vi "TestCloneAPI.vi"() -> ()   [LabVIEW 2018, in "AcPwrModule.lvlib"]
uses:
  AcPwrModule.lvlib
  AcPwrPlugins/ChromaAcLoad/TypeDefs/DeviceProperties.ctl
  TestInfo.ctl
  <userlib>/NIST/ModuleAdminLib/CloneRegistration/CloneRegistration.lvclass
  <userlib>/NIST/ModuleAdminLib/ModuleAdmin/ModuleAdmin.lvclass/ModuleAdmin.ctl
  <userlib>/NIST/ModuleAdminLib/ModuleAdmin/ModuleAdmin.lvclass
  PublicAPI/Arguments/Broadcasts/clDidInit.ctl
  PublicAPI/Arguments/Requests/clStopArgument.ctl
  <userlib>/NIST/ModuleAdminLib/ModuleAdmin/Accessors/Read CloneRegRef.vi
  <userlib>/NIST/ModuleAdminLib/ModuleAdmin/Accessors/Write CloneRegRef.vi
  AcPwrPlugins/AcPwrBaseClass/AcPwrBase.lvclass
  Visualization/Visualization.lvlib
  AcPwrPlugins/ChromaAcLoad/ChromaAcLoad.lvclass
panel:
  in  "Cluster":T1 {"Phases"."Phase Select" items=["Phase ALL", "Phase A", "Phase B", "Phase C"]}
  in  "btnSet":bool
  in  "btnGet":bool
  in  "btnVisualize":bool
  in  "Tab Control":enum32{"AC", "DC"}(tab)
  out "PacificPower":waveform(dbl)[](graph) caption="4140002"
  out "PP Incorrect Data Type?":bool
  out "Chroma AC":waveform(dbl)[](graph) caption="4140002"
  out "Chroma AC Incorrect Data Type?":bool
  out "NHRDC":waveform(sgl)[](graph) caption="4140002"
  out "NHRDC Incorrect Data Type?":bool
  out "Chroma DC":waveform(dbl)[](graph) caption="4140002"
  out "Chroma DC Incorrect Data Type?":bool
  in  "PP Program Number":i32=1 min=1 max=99
  in  "btnInitialize":bool
  in  "btnClearStatusLog":bool
  in  "btnDeviceOff":bool
  in  "btnDeviceOn":bool
  in  "btnConfigDevice":bool caption="btnConfigDevices"
  in  "btnStartMeas":bool
  in  "btnStopMeas":bool
  in  "btnClose":bool
  in  "btnReset":bool
  in  "btnPref":bool
  in  "Show Panel":bool
  in  "Plugin Type":u16(ring) items=["AcPwrBase", "ChromaDCLoad", "ChromaACLoad", "NHRDCPower", "PPS360AMXT"]
  in  "btnLoadPlugin":bool
  out "Path":path
  in  "btnRequestINIPath":bool
  in  "btnRemove":bool
  out "Status Log":string
  out "Active Modules (Array)":string[](array[string])
  in  "btnAdd":bool
  in  "btnStop":bool
  in  "Select Module":i32(ring)=-1 caption="Select Module to send Request" items=["All"=-1]
  # "Measurements"
  # "Hidden"
  # "Visible"
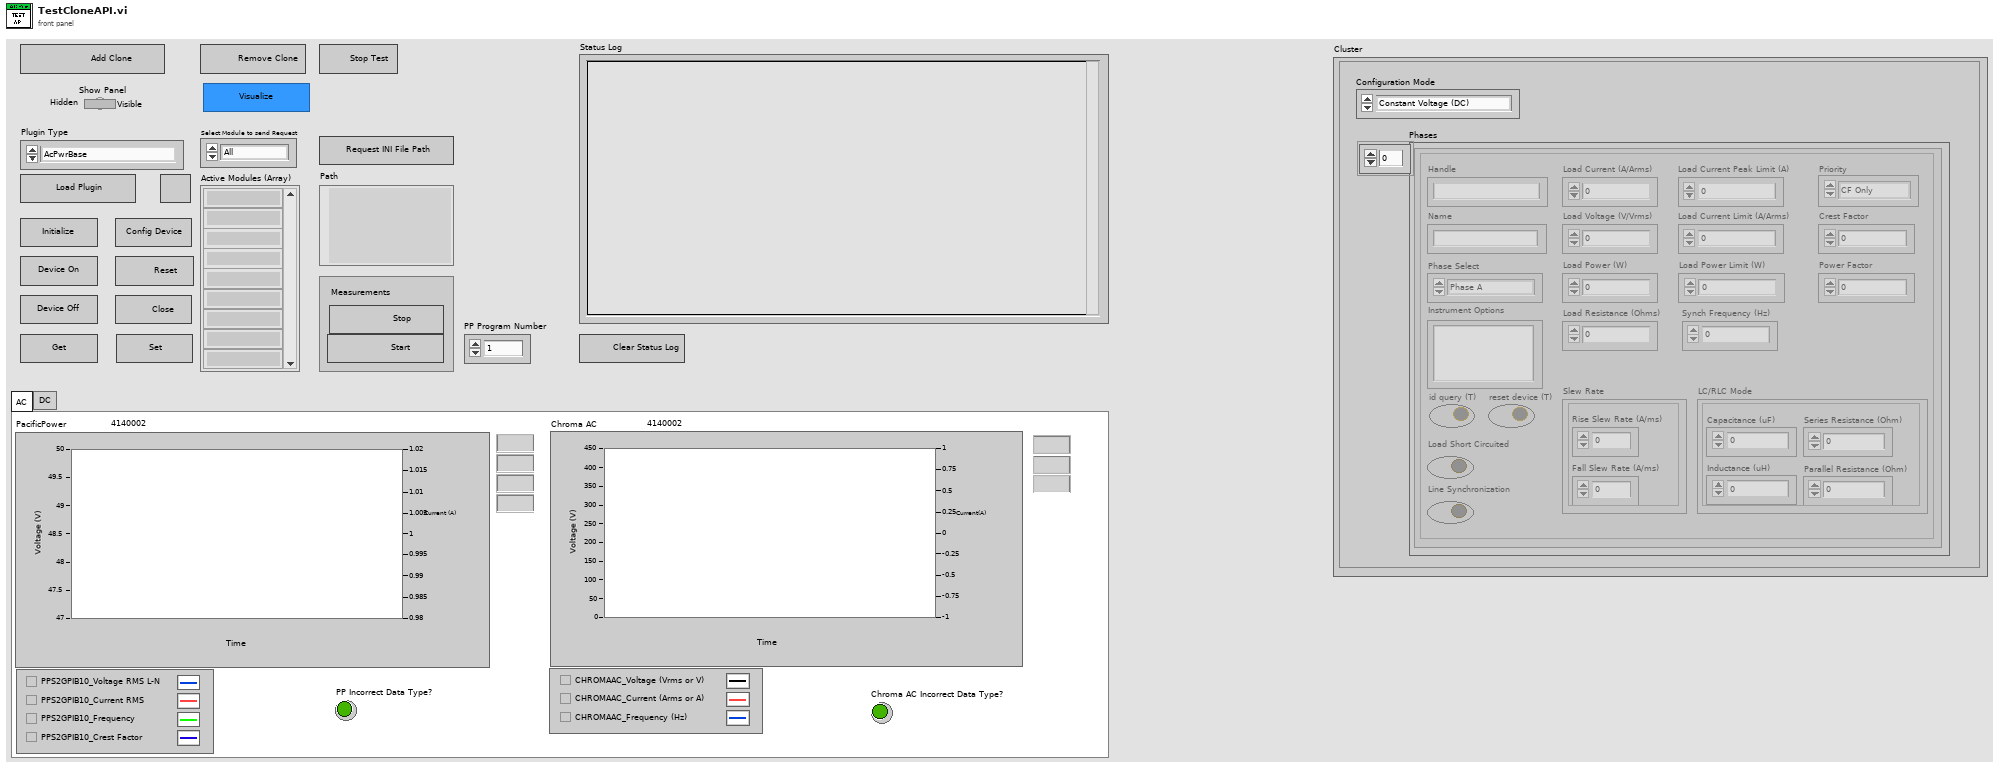
[diagram p1: front panel]
types:
  T1 = typedef "AcPwrPlugins.lvlib/ChromaAcLoad.lvclass/DeviceProperties.ctl" = cluster{"Configuration Mode":enum16{"Constant Voltage (DC)", "Constant Power (DC)", "Constant Power (AC)", "Constant Current (DC)", "Constant Current (AC)", "Constant Resistance (DC)", "Constant Resistance (AC)", "Rectified Mode (DC)", "Inrush (AC)", "RLC CP (AC)", "RLC (AC)"}, "Phases":cluster{"Handle":string, "Name":string, "Phase Select":i32, "Instrument Options":string, "id query (T)":bool, "reset device (T)":bool, "Load Short Circuited":bool, "Line Synchronization":bool, "Load Current (A/Arms)":dbl, "Load Voltage (V/Vrms)":dbl, "Load Power (W)":dbl, "Load Resistance (Ohms)":dbl, "Load Current Peak Limit (A)":dbl, "Load Current Limit (A/Arms)":dbl, "Load Power Limit (W)":dbl, "Synch Frequency (Hz)":dbl, "Priority":enum16{"CF Only", "PF Only", "Both (CF)", "Both (PF)"}, "Crest Factor":dbl, "Power Factor":dbl, "Slew Rate":cluster{"Rise Slew Rate (A/ms)":i32, "Fall Slew Rate (A/ms)":i32}, "LC/RLC Mode":cluster{"Capacitance (uF)":i32, "Inductance (uH)":i32, "Series Resistance (Ohm)":dbl, "Parallel Resistance (Ohm)":dbl}, "Timing":cluster{"TimingOn":enum16{""}, "Hours":u32, "Minutes":u32, "Seconds":dbl, "CutoffVoltage":dbl}, "Connected":bool}[]}
  T2 = typedef "AcPwrModule.lvlib/TestInfo.ctl" = cluster{"PluginIniFilePaths":path[]}
  T3 = typedef "AcPwrModule.lvlib/clBroadcastEvents.ctl" = cluster{"DidInit":refnum<user-event>, "StatusUpdate":refnum<user-event>, "ErrorReport":refnum<user-event>, "DidStop":refnum<user-event>, "PathToINI":refnum<user-event>, "Measurements":refnum<user-event>, "LoadConfigFile":refnum<user-event>, "GetSettings":refnum<user-event>, "SetSettings":refnum<user-event>, "GetType&ID":refnum<user-event>}
  T4 = typedef "AcPwrModule.lvlib/clDidInit.ctl" = cluster{"Init?":bool, "ModuleAdmin":refnum<class "ModuleAdmin.lvclass">}
  T5 = typedef "AcPwrModule.lvlib/clStopArgument.ctl" = cluster{"Exit via Stop Module Req?":bool, "Wait for Module to stop?":bool, "ModuleAdmin":refnum<class "ModuleAdmin.lvclass">}
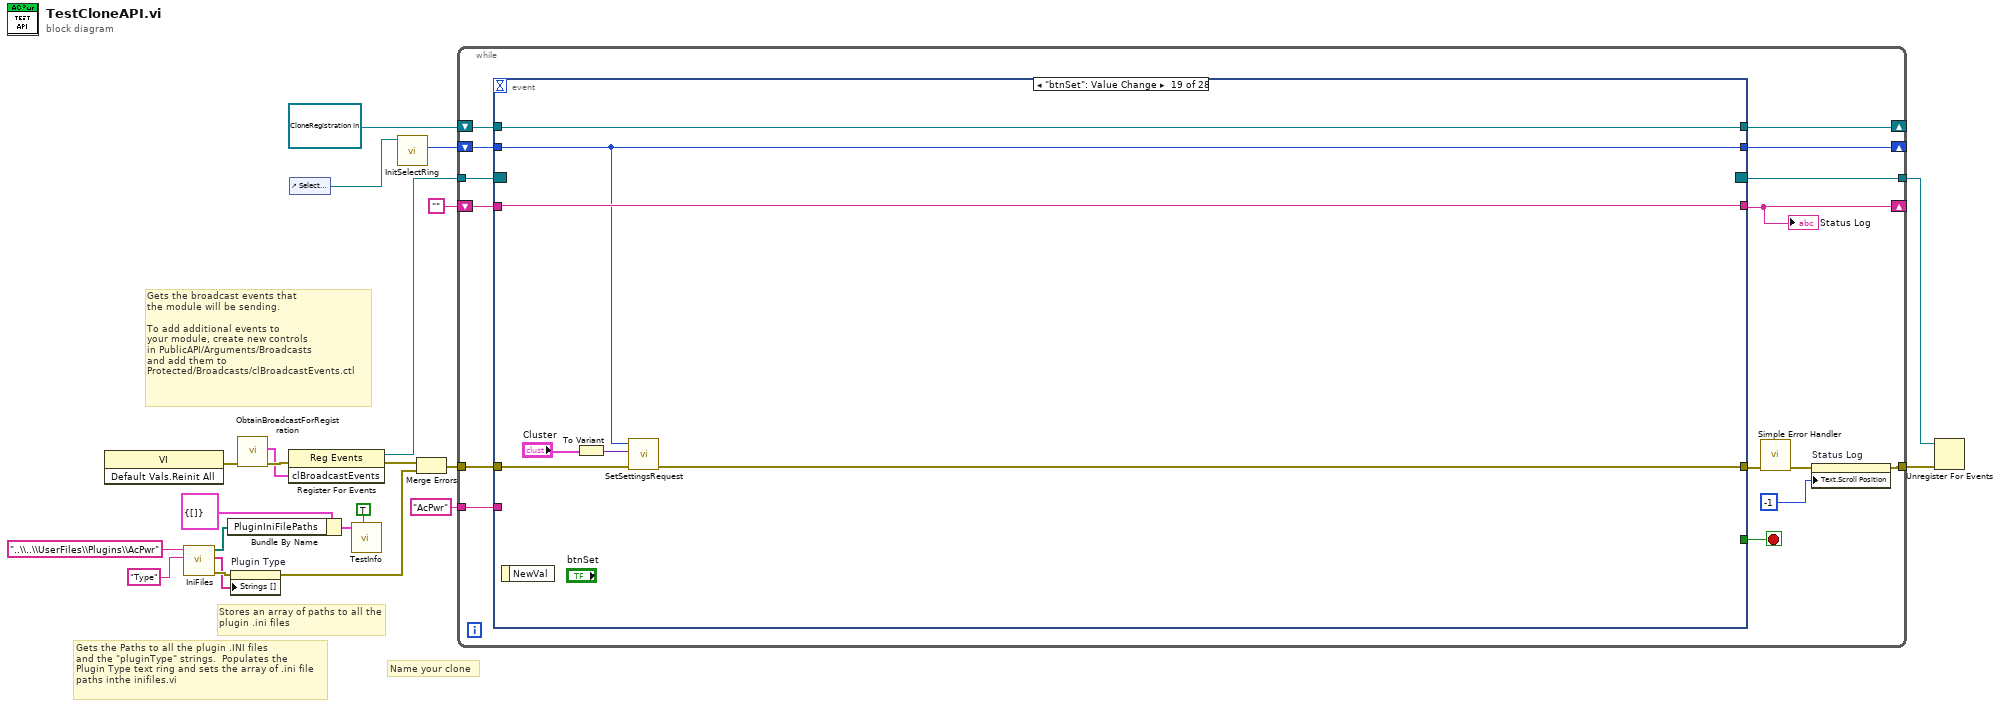
[diagram p0: block diagram]
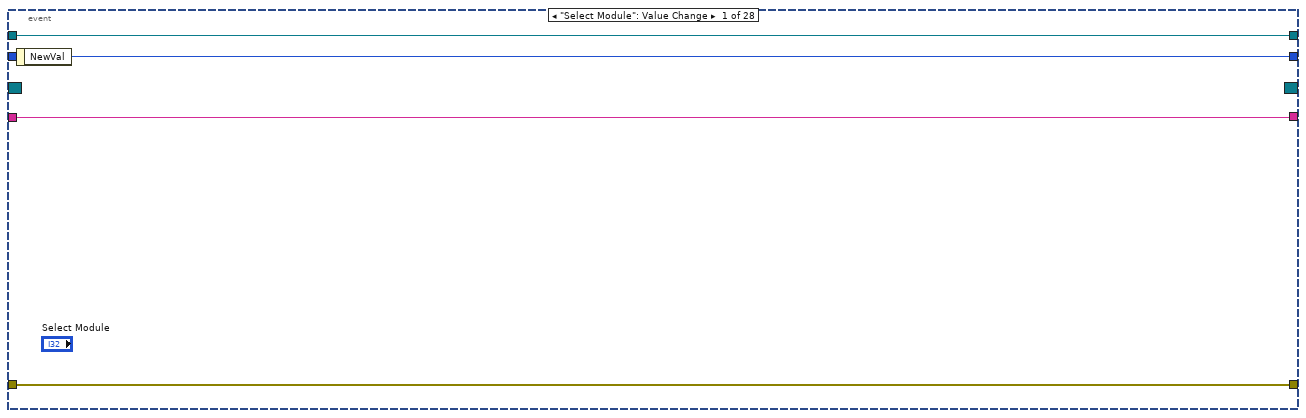
[diagram p2: hidden frame]
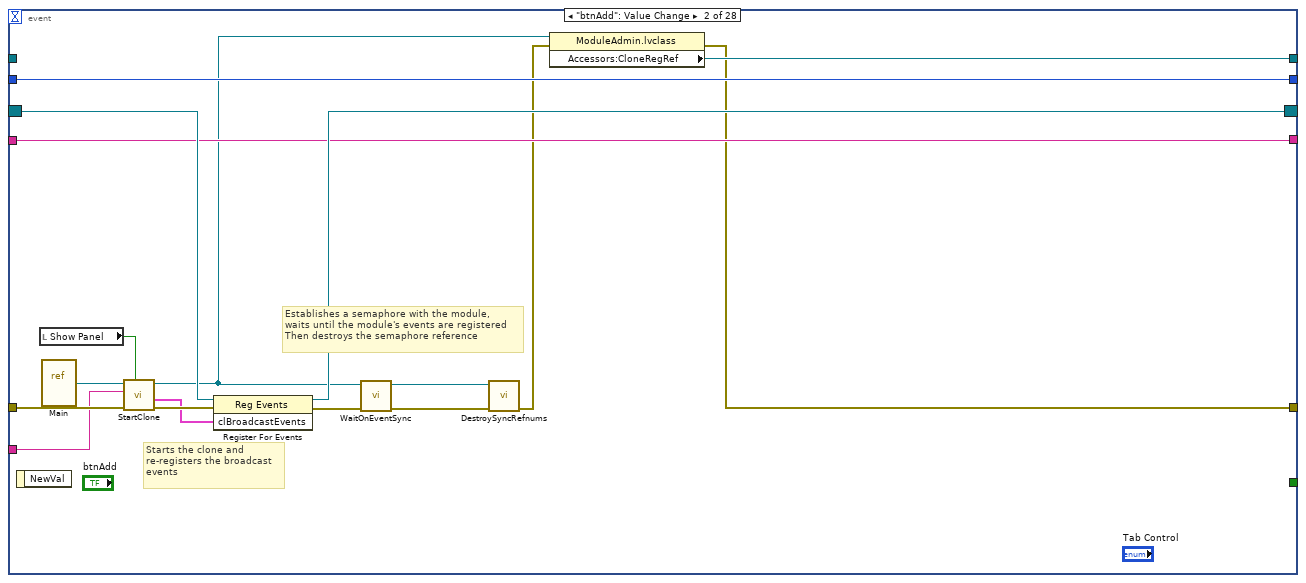
[diagram p3: hidden frame]
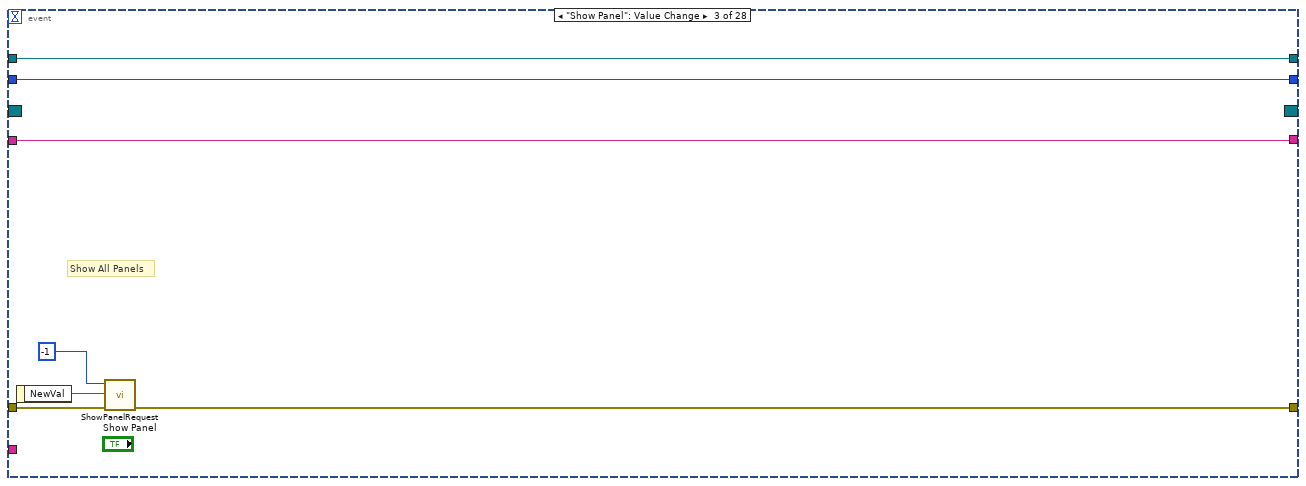
[diagram p4: hidden frame]
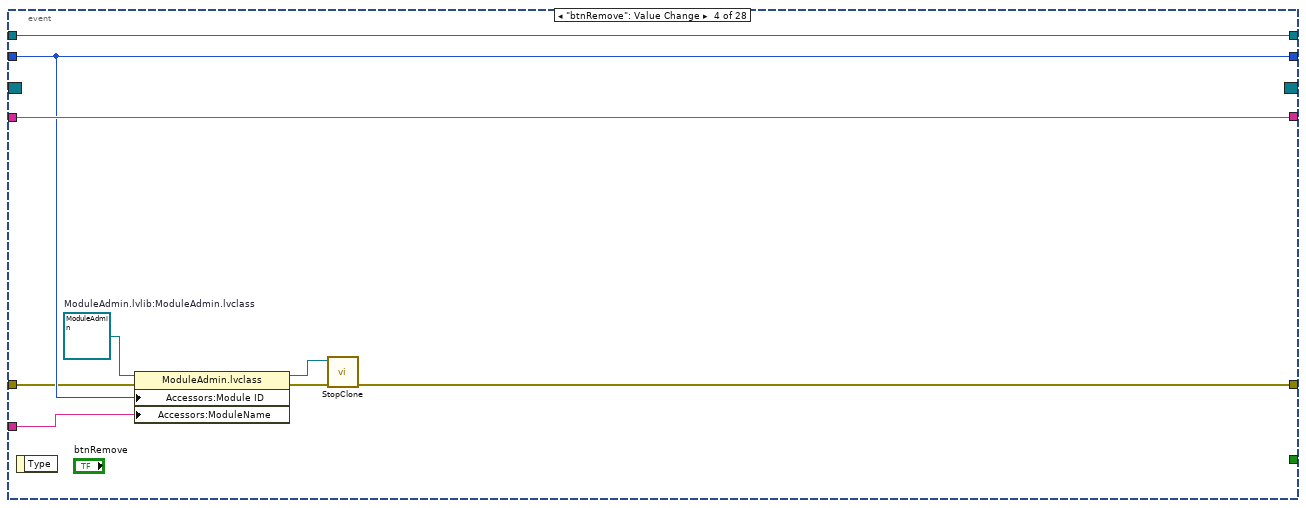
[diagram p5: hidden frame]
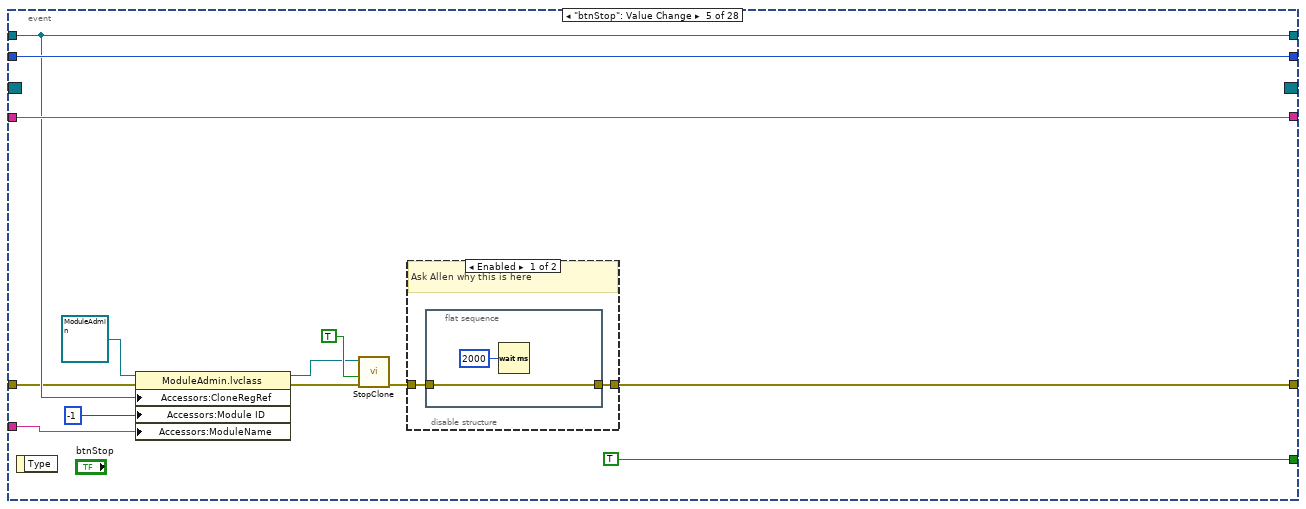
[diagram p6: hidden frame]
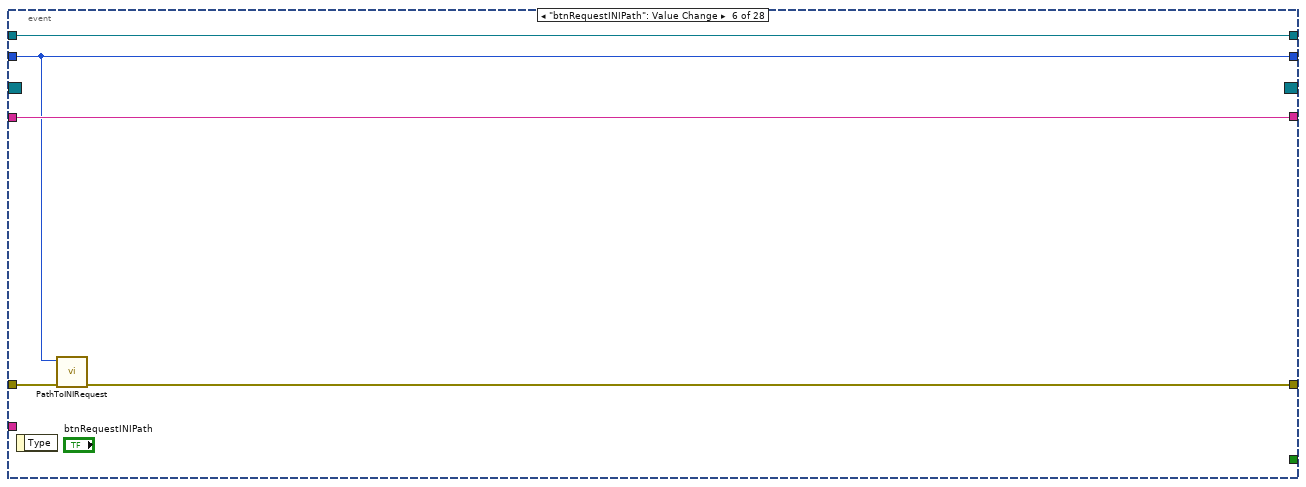
[diagram p8: hidden frame]
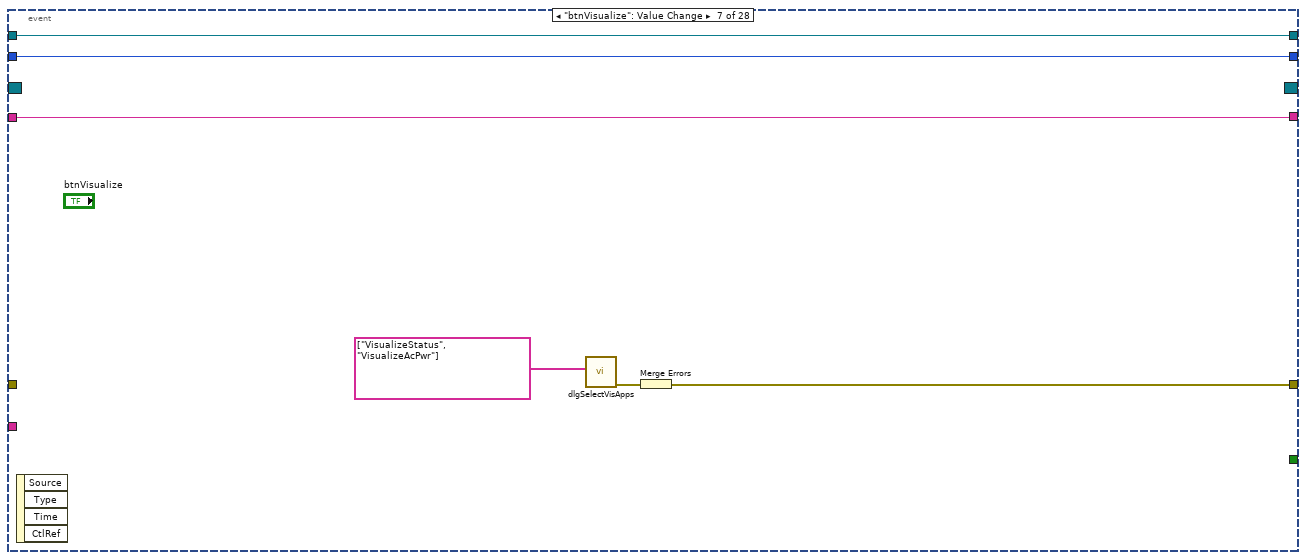
[diagram p9: hidden frame]
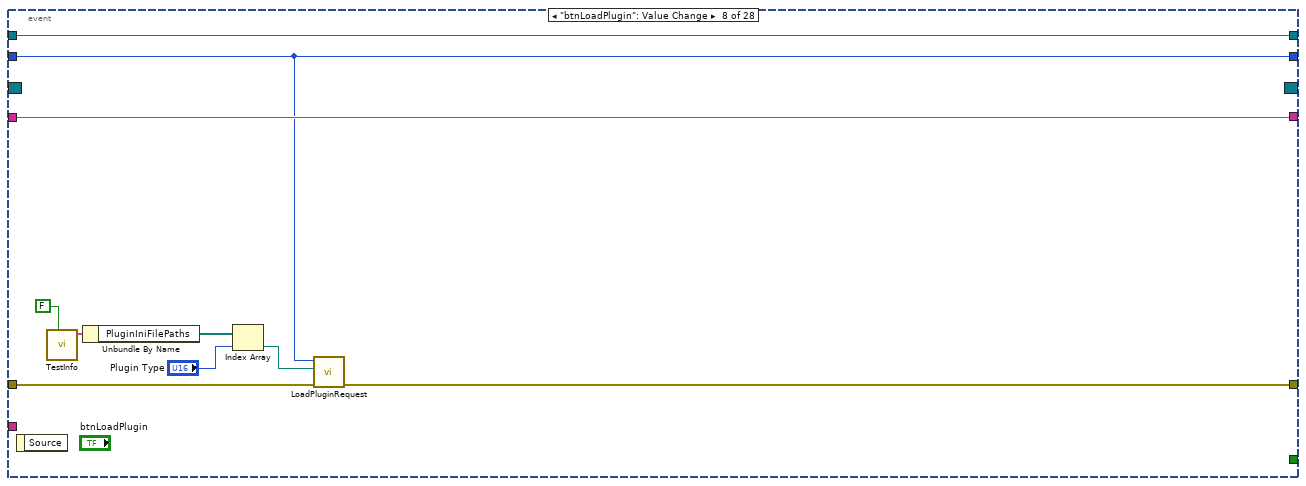
[diagram p10: hidden frame]
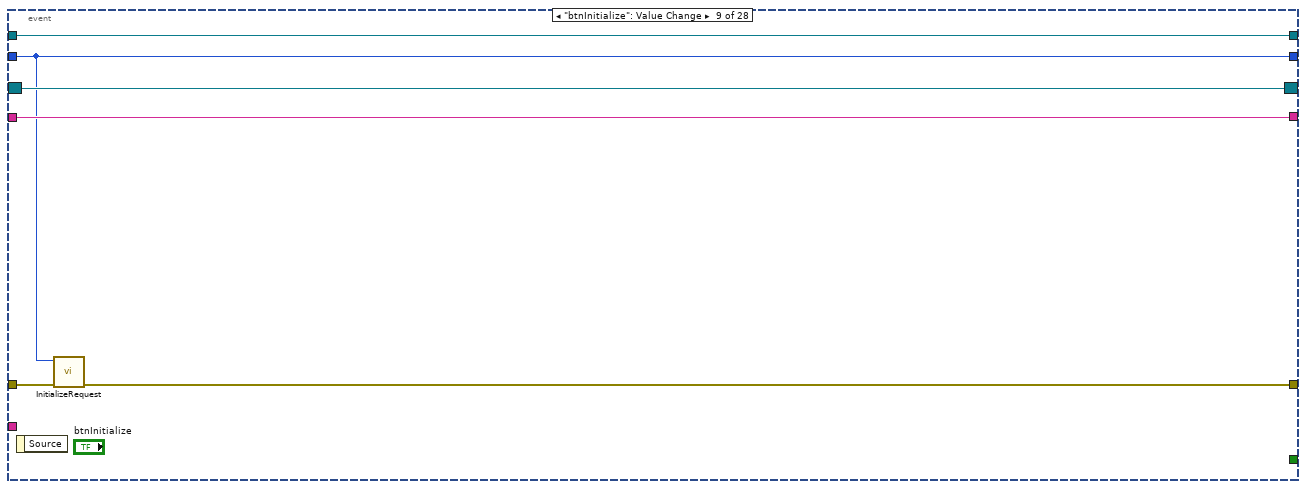
[diagram p11: hidden frame]
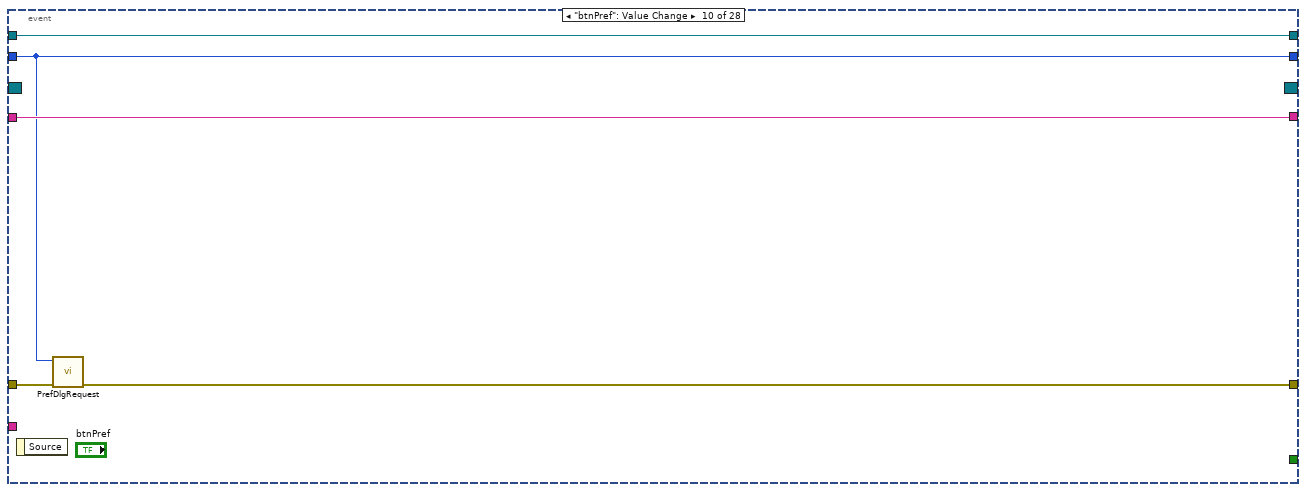
[diagram p12: hidden frame]
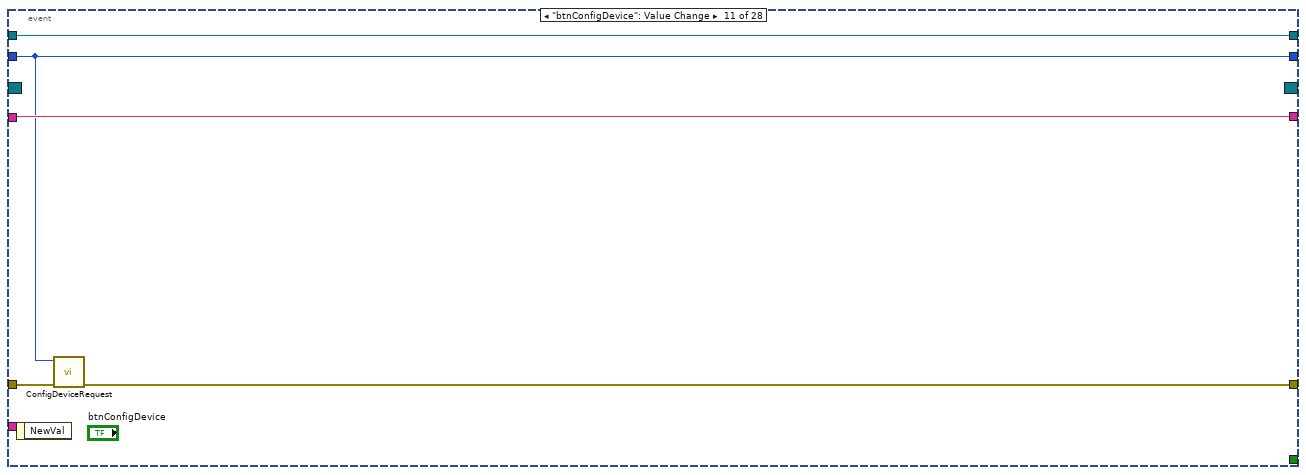
[diagram p13: hidden frame]
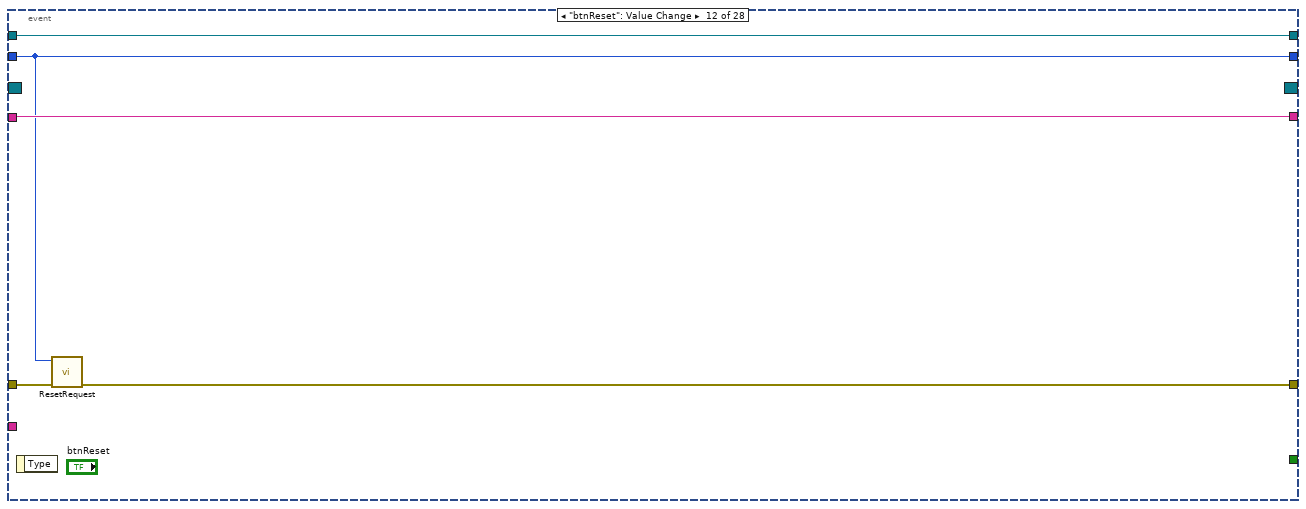
[diagram p14: hidden frame]
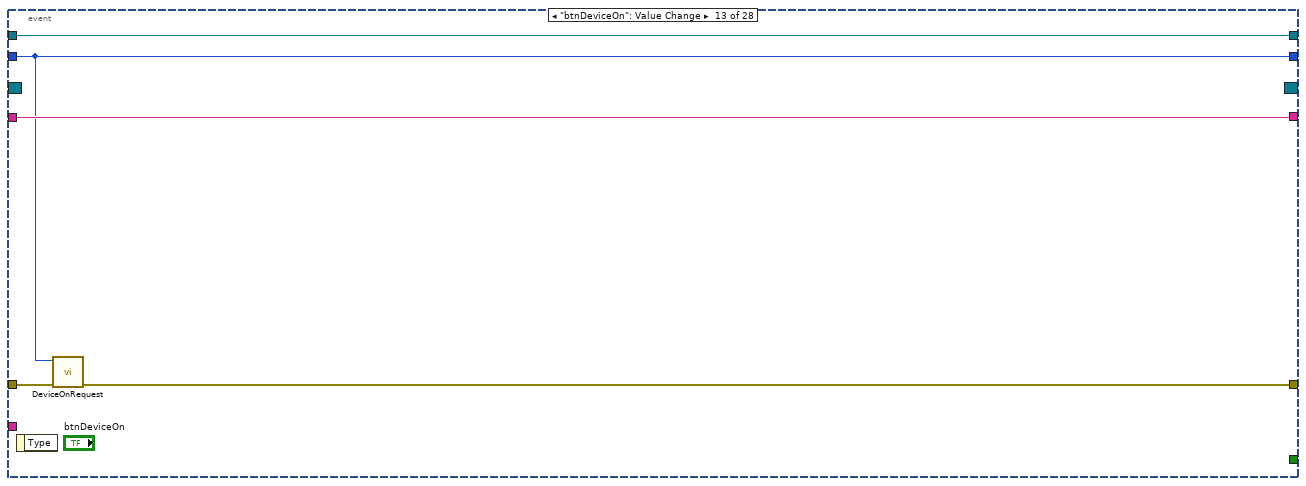
[diagram p15: hidden frame]
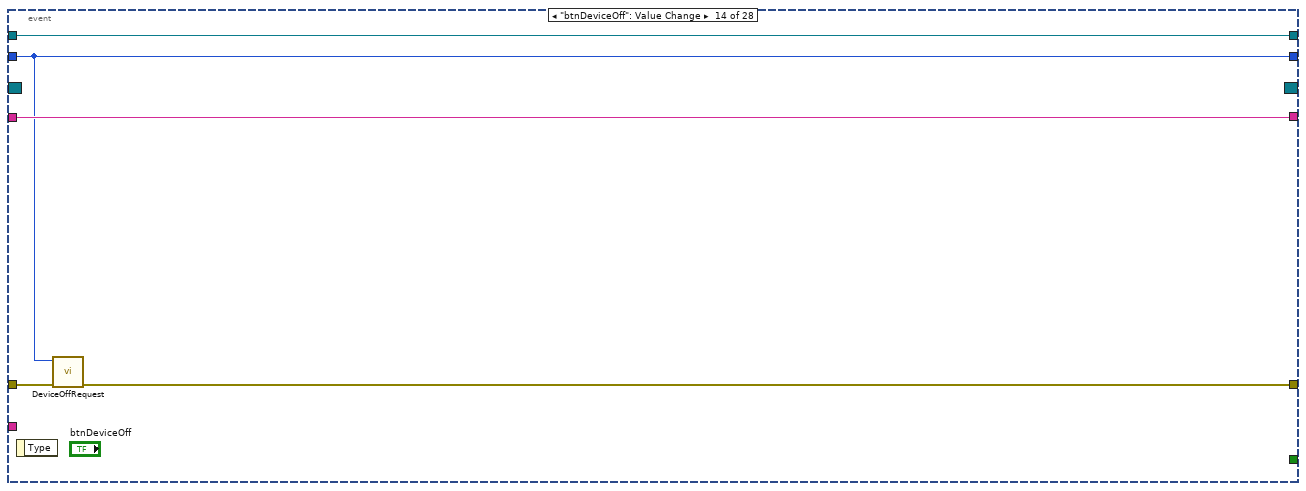
[diagram p16: hidden frame]
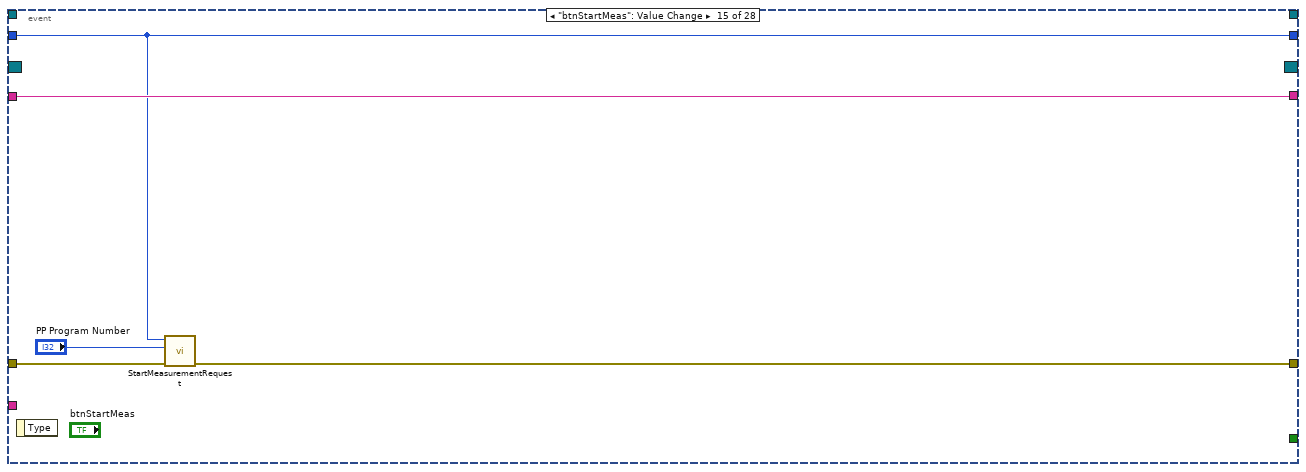
[diagram p17: hidden frame]
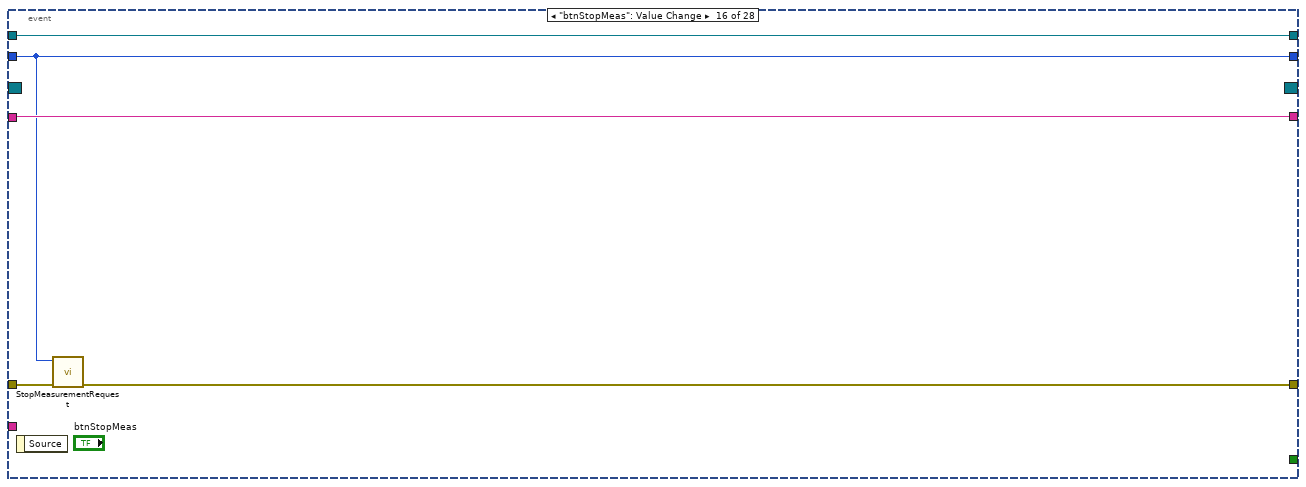
[diagram p18: hidden frame]
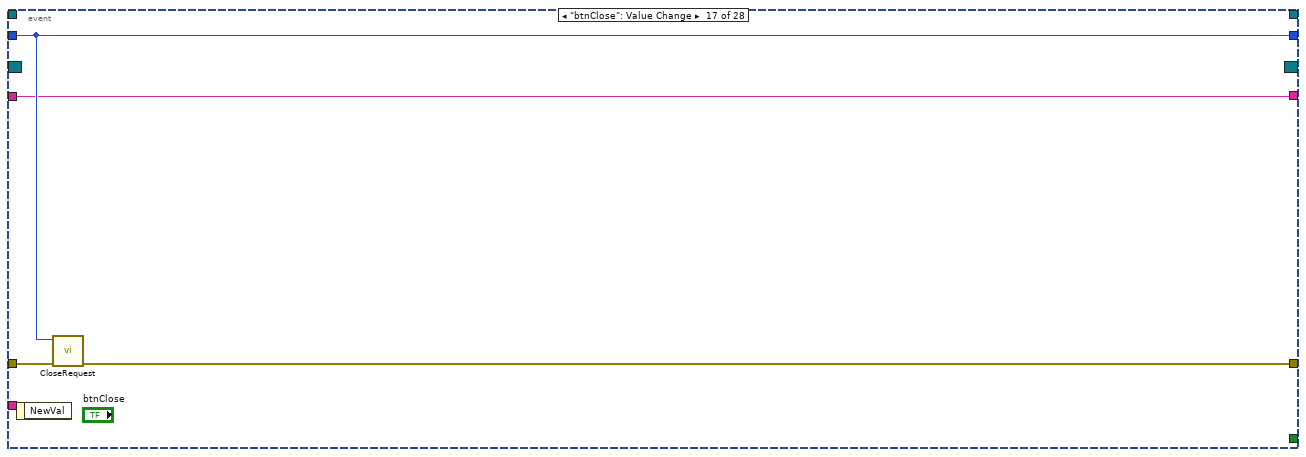
[diagram p19: hidden frame]
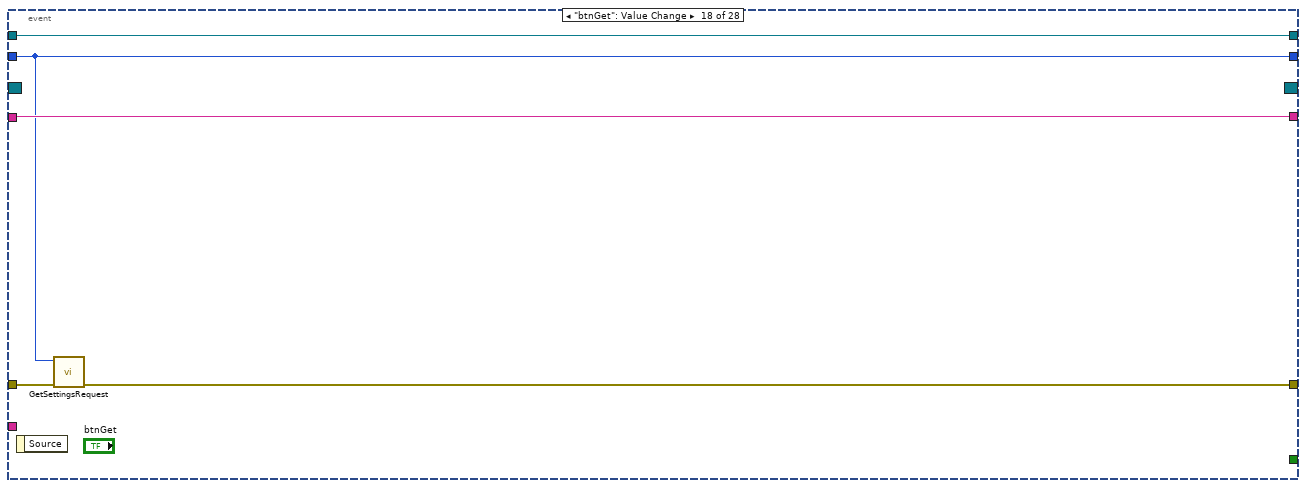
[diagram p20: hidden frame]
diagram:
  # "Stores an array of paths to all the plugin .ini files"
  # "Gets the Paths to all the plugin .INI files\nand the \"pluginType\" strings.  Populates the \nPlugin Type text ring and sets the array of .ini file\npaths inthe inifiles.vi"
  # "Name your clone"
  # "Gets the broadcast events that\nthe module will be sending.\n\nTo add additional events to\nyour module, create new controls\nin PublicAPI/Arguments/Broadcasts\nand add them to\nProtected/Broadcasts/clBroadcastEvents.ctl"
  n1 = invoke class="VI" method="Default Vals.Reinit All"() -> (error out=w20:errorcluster)  [unwired: 3 in, 2 out]
  n2 = call "IniFiles.vi"("iniKey"="Type", "name or relative path"="..\\..\\UserFiles\\Plugins\\AcPwr") -> ("error out"=w13:errorcluster, "Types"=w12:string[], "IniFilePaths"=w11:path[])  [unwired: 7 in]
  n3 = Bundle By Name(cluster=T2 {"PluginIniFilePaths"=[]} ("TestInfo"), "PluginIniFilePaths"=w11) -> (w10:T2)
  n4 = property on="Plugin Type" class="Ring (strict)"(error in=w13, "Strings []"=w12) -> (error out=w7:errorcluster)  [unwired: 1 in, 1 out]
  n5 = call "ObtainBroadcastForRegistration.vi"("error in (no error)"=w20) -> ("error out"=w19:errorcluster, "clBroadcastEvents"=w18:T3)  [unwired: 9 in]
  n6 = register-events(error in=w19, w18) -> (reference out=w16:refnum<event-registration>, error out=w17:errorcluster)  [unwired: 1 in]
  n7 = control-ref of="Select Module"() -> (w22:refnum<vi>)
  n8 = call "TestInfo.vi"("Set (f)"=TRUE, "TestInfo 2"=w10) -> ()  [unwired: 9 in, 1 out]
  n9 = call "InitSelectRing.vi"("Ring Refnum"=w22) -> ("Module Ring Value"=w21:i32)  [unwired: 9 in, 1 out]
  n10 = Merge Errors(w17, w7) -> (w8:errorcluster)
  n11 = while {
    shift-right: [w36] -> _
    shift-left: w21 -> [w37]
    tunnel: w8 -> [w34]
    tunnel: w16 -> [w32]
    tunnel: [w24] -> w3
    shift-right: [w31] -> _
    shift-left: "" -> [w30]
    tunnel: "AcPwr" ("ModuleName") -> [w29]
    tunnel: [w28] -> w2
    shift-right: [w27] -> _
    shift-left: refnum<data-value> refnum ("Accessors:CloneRegRef") -> [w26]
    stop <- w35 stop-if-true
    n12 = event shown="[18] \"btnSet\": Value Change" {
      selector: w32 -> [_ w51 _ _ _ _ _ _ w119 _ _ _ _ _ _ _ _ _ _ _ _ _ _ _ _ _ _ _]
      dyn-events: [_ w50 _ _ _ _ _ _ w119 _ _ _ _ _ _ _ _ _ _ _ _ _ _ _ _ _ _ _] -> w28
      timeout: _ -> [_ _ _ _ _ _ _ _ _ _ _ _ _ _ _ _ _ _ _ _ _ _ _ _ _ _ _ _]
      tunnel: w37 -> [_ w58 w61 w71 w87 w96 w102 w110 w114 w123 w126 w130 w135 w141 w146 w152 w158 w160 w164 w173 _ _ w236 w245 w294 w298 w311 w340]
      tunnel: [w41 w58 w61 w71 w87 w96 w102 w110 w114 w123 w126 w130 w135 w141 w146 w152 w158 w160 w164 w173 w194 w210 w236 w245 w294 w298 w311 w340] -> w36
      tunnel: [_ _ _ _ TRUE _ _ _ _ _ _ _ _ _ _ _ _ _ _ _ _ _ _ _ _ _ _ _] -> w35
      tunnel: w34 -> [w39 w57 w64 w66 w76 w95 _ w112 w115 w122 w128 w131 w139 w144 w149 w150 w157 w161 w166 w171 w198 w218 w233 w243 w258 w303 w307 w316]
      tunnel: [w39 w42 w62 w73 w77 w94 w99 w111 w116 w121 w125 w132 w136 w140 w147 w151 w156 w159 w167 w171 w185 w209 w223 w240 w293 w302 w306 w324] -> w33
      tunnel: [w40 w48 w60 w74 w84 w97 w101 w113 w117 w124 w127 w133 w138 w143 w148 w154 w155 w163 w170 "" w187 w215 w229 w244 w270 w297 w312 w323] -> w31
      tunnel: w30 -> [w40 w48 w60 w74 w84 w97 w101 w113 w117 w124 w127 w133 w138 w143 w148 w154 w155 w163 w170 _ w186 w216 w235 w244 w274 w297 w312 w325]
      tunnel: w29 -> [_ w47 _ w70 w82 _ _ _ _ _ _ _ _ _ _ _ _ _ _ _ _ _ _ _ _ _ _ _]
      tunnel: [w38 w45 w59 w68 w79 w93 w103 w104 w118 w120 w129 w134 w137 w142 _ w153 _ w162 w169 w174 w179 w202 w224 w241 _ w295 w305 w341] -> w27
      tunnel: w26 -> [w38 _ w59 w68 w79 w93 w103 w104 w118 w120 w129 w134 w137 w142 _ w153 _ w162 w169 w174 w179 w202 w224 w241 _ w295 w305 w341]
      event "Select Module": Value Change {
        n13 = event-data() -> ("NewVal"=w41:i32)  [unwired: 1 in]
      }
      event "btnAdd": Value Change {
        # "Establishes a semaphore with the module,\nwaits until the module's events are registered\nThen destroys the semaphore reference"
        # "Starts the clone and\nre-registers the broadcast \nevents"
        n14 = event-data() -> ()  [unwired: 1 in, 1 out]
        n15 = local read "Show Panel"() -> (w44:bool)
        n16 = vi-ref "Main.vi"() -> (w49:refnum<vi>)
        n17 = call "StartClone.vi"("ShowPanel? (f)"=w44, "error in (no error)"=w57, "ModuleName"=w47, "VI Refnum"=w49) -> ("error out"=w56:errorcluster, "clBroadcastEvents"=w52:T3, "ModuleAdmin"=w46:refnum<class "ModuleAdmin.lvclass">)  [unwired: 5 in]
        n18 = register-events(reference=w51, error in=w56, w52) -> (reference out=w50:refnum<event-registration>, error out=w55:errorcluster)
        n19 = call <userlib>:"WaitOnEventSync.vi"("error in (no error)"=w55, "ModuleAdmin"=w46) -> ("error out"=w54:errorcluster, "ModuleAdmin"=w53:refnum<class "ModuleAdmin.lvclass">)  [unwired: 8 in]
        n20 = call <userlib>:"DestroySyncRefnums.vi"("error in (no error)"=w54, "ModuleAdmin"=w53) -> ("error out"=w43:errorcluster)  [unwired: 9 in]
        n21 = property class="ModuleAdmin.lvclass"(reference=w46, error in=w43) -> (error out=w42:errorcluster, "Accessors:CloneRegRef"=w45:refnum<data-value>)  [unwired: 1 out]
      }
      event "Show Panel": Value Change {
        # "Show All Panels"
        n22 = event-data() -> ("NewVal"=w65:bool)  [unwired: 1 in]
        n23 = call "ShowPanelRequest.vi"("error in (no error)"=w64, "ShowPanel?"=w65, "ModuleID"=-1) -> ("error out"=w62:errorcluster)  [unwired: 8 in]
      }
      event "btnRemove": Value Change {
        w72 = refnum<class "ModuleAdmin.lvclass"> refnum  # ModuleAdmin.lvlib:ModuleAdmin.lvclass
        n24 = event-data() -> ()  [unwired: 1 in, 1 out]
        n25 = property class="ModuleAdmin.lvclass"(reference=w72, error in=w66, "Accessors:Module ID"=w71, "Accessors:ModuleName"=w70) -> (reference out=w69:refnum<class "ModuleAdmin.lvclass">, error out=w67:errorcluster)
        n26 = call "StopClone.vi"("error in (no error)"=w67, "ModuleAdmin"=w69) -> ("error out"=w73:errorcluster)  [unwired: 9 in]
      }
      event "btnStop": Value Change {
        n27 = event-data() -> ()  [unwired: 1 in, 1 out]
        n28 = property class="ModuleAdmin.lvclass"(reference=refnum<class "ModuleAdmin.lvclass"> refnum ("ModuleAdmin.lvlib:ModuleAdmin.lvclass"), error in=w76, "Accessors:CloneRegRef"=w79, "Accessors:Module ID"=-1 ("Module ID"), "Accessors:ModuleName"=w82) -> (reference out=w81:refnum<class "ModuleAdmin.lvclass">, error out=w75:errorcluster)
        n29 = call "StopClone.vi"("error in (no error)"=w75, "Wait for Module to stop?"=TRUE, "ModuleAdmin"=w81) -> ("error out"=w78:errorcluster)  [unwired: 8 in]
        n30 = disable-structure "Diagram Disable Structure" shown="Enabled" {
          disable-tunnel: w78 -> [w89 w92]
          disable-tunnel: [w88 w92] -> w77
          frame Enabled {
            # "Ask Allen why this is here"
            n31 = flat-sequence {
              tunnel: w89 -> [w90]
              tunnel: [w90] -> w88
              frame #0 {
                n32 = Wait (ms)(milliseconds to wait=u32 2000) -> ()  [unwired: 1 out]
              }
            }
          }
          frame Disabled {
          }
        }
      }
      event "btnRequestINIPath": Value Change {
        n33 = event-data() -> ()  [unwired: 1 in, 1 out]
        n34 = call "PathToINIRequest.vi"("error in (no error)"=w95, "ModuleID"=w96) -> ("error out"=w94:errorcluster)  [unwired: 9 in]
      }
      event "btnVisualize": Value Change {
        n35 = event-data() -> ()  [unwired: 1 in, 4 out]
        n36 = call "dlgSelectVisApps.vi"("PathsToVisApps"=string[] ["VisualizeStatus", "VisualizeAcPwr"]) -> ("Error Out"=w100:errorcluster[])  [unwired: 10 in]
        n37 = Merge Errors(w100) -> (w99:errorcluster)
      }
      event "btnLoadPlugin": Value Change {
        n38 = event-data() -> ()  [unwired: 1 in, 1 out]
        n39 = call "TestInfo.vi"("Set (f)"=FALSE) -> ("TestInfo"=w108:T2)  [unwired: 10 in]
        n40 = Unbundle By Name(w108) -> ("PluginIniFilePaths"=w107:path[])
        n41 = Index Array(array=w107, index="Plugin Type") -> (element=w105:path)
        n42 = call "LoadPluginRequest.vi"("error in (no error)"=w112, "PathToPluginINI"=w105, "ModuleID"=w110) -> ("error out"=w111:errorcluster)  [unwired: 8 in]
      }
      event "btnInitialize": Value Change {
        n43 = event-data() -> ()  [unwired: 1 in, 1 out]
        n44 = call "InitializeRequest.vi"("error in (no error)"=w115, "ModuleID"=w114) -> ("error out"=w116:errorcluster)  [unwired: 9 in]
      }
      event "btnPref": Value Change {
        n45 = event-data() -> ()  [unwired: 1 in, 1 out]
        n46 = call "PrefDlgRequest.vi"("error in (no error)"=w122, "ModuleID"=w123) -> ("error out"=w121:errorcluster)  [unwired: 9 in]
      }
      event "btnConfigDevice": Value Change {
        n47 = event-data() -> ()  [unwired: 1 in, 1 out]
        n48 = call "ConfigDeviceRequest.vi"("Error In"=w128, "ModuleID"=w126) -> ("Error Out"=w125:errorcluster)  [unwired: 9 in]
      }
      event "btnReset": Value Change {
        n49 = event-data() -> ()  [unwired: 1 in, 1 out]
        n50 = call "ResetRequest.vi"("Error In"=w131, "ModuleID"=w130) -> ("Error Out"=w132:errorcluster)  [unwired: 9 in]
      }
      event "btnDeviceOn": Value Change {
        n51 = event-data() -> ()  [unwired: 1 in, 1 out]
        n52 = call "DeviceOnRequest.vi"("Error In"=w139, "ModuleID"=w135) -> ("Error Out"=w136:errorcluster)  [unwired: 9 in]
      }
      event "btnDeviceOff": Value Change {
        n53 = event-data() -> ()  [unwired: 1 in, 1 out]
        n54 = call "DeviceOffRequest.vi"("Error In"=w144, "ModuleID"=w141) -> ("Error Out"=w140:errorcluster)  [unwired: 9 in]
      }
      event "btnStartMeas": Value Change {
        n55 = event-data() -> ()  [unwired: 1 in, 1 out]
        n56 = call "StartMeasurementRequest.vi"("Error In"=w149, "Program Number"="PP Program Number", "ModuleID"=w146) -> ("Error Out"=w147:errorcluster)  [unwired: 8 in]
      }
      event "btnStopMeas": Value Change {
        n57 = event-data() -> ()  [unwired: 1 in, 1 out]
        n58 = call "StopMeasurementRequest.vi"("Error In"=w150, "ModuleID"=w152) -> ("Error Out"=w151:errorcluster)  [unwired: 9 in]
      }
      event "btnClose": Value Change {
        n59 = event-data() -> ()  [unwired: 1 in, 1 out]
        n60 = call "CloseRequest.vi"("error in (no error)"=w157, "ModuleID"=w158) -> ("error out"=w156:errorcluster)  [unwired: 9 in]
      }
      event "btnGet": Value Change {
        n61 = event-data() -> ()  [unwired: 1 in, 1 out]
        n62 = call "GetSettingsRequest.vi"("Error In"=w161, "ModuleID"=w160) -> ("Error Out"=w159:errorcluster)  [unwired: 9 in]
      }
      event "btnSet": Value Change {
        n63 = event-data() -> ()  [unwired: 1 in, 1 out]
        n64 = To Variant(anything="Cluster") -> (Variant=w165:variant)
        n65 = call "SetSettingsRequest.vi"("Error In"=w166, "Data"=w165, "ModuleID"=w164) -> ("Error Out"=w167:errorcluster)  [unwired: 8 in]
      }
      event "btnClearStatusLog": Value Change {
        n66 = event-data() -> ()  [unwired: 1 in, 1 out]
      }
      event User Event {
        # "Adds the module ID to the \nSelect Module ring"
        # "Time stamp and add the DidInit message to the log"
        # "The data types for the broadcast messages\nare in PublicAPI/Broadcasts"
        n67 = event-data() -> ("Data"=w197:variant)  [unwired: 1 in]
        n68 = Variant To Data(error in=w198, type=T4 {"Init?"=FALSE, "ModuleAdmin"=refnum} ("clDidInit"), Variant=w197) -> (data=w191:T4, error out=w175:errorcluster)
        n69 = Unbundle By Name(w191) -> ("ModuleAdmin"=w183:refnum<class "ModuleAdmin.lvclass">)
        n70 = property class="ModuleAdmin.lvclass"(reference=w183, error in=w175) -> (error out=w177:errorcluster, "Accessors:ModuleName"=w181:string, "Accessors:Module ID"=w180:i32, "Accessors:CloneRegRef"=w178:refnum<data-value>)  [unwired: 1 out]
        n71 = Get Date/Time In Seconds() -> (seconds since 1Jan1904=w189:timestamp)
        n72 = Get Date/Time String(date format (0)=enum16{"short", "long", "abbreviated"}."short", seconds (now)=w189, want seconds? (F)=TRUE) -> (time string=w192:string)  [unwired: 1 out]
        n73 = control-ref of="Select Module"() -> (w195:refnum<vi>)
        n74 = Format Into String(format string="%s: %s %d%s \\r", initial string=w186, error in=w177, w192, w181, w180, ": The clone has initialized successfully. ") -> (resulting string=w187:string, error out=w176:errorcluster)
        n75 = call "UpdateSelectRing.vi"("error in (no error)"=w176, "CloneRegRef"=w178, "Ring Refnum"=w195) -> ("error out"=w185:errorcluster, "ActiveModules"=→"Active Modules (Array)":string[], "Module Ring Value"=w194:i32)  [unwired: 6 in]
      }
      event User Event {
        # "Time stamp and add the Stop message to the log"
        # "The Stop Argument  is found in\nPublicAPI/Arguments/Requests"
        n76 = event-data() -> ("Data"=w217:variant)  [unwired: 1 in]
        n77 = Variant To Data(error in=w218, type=T5 {"Exit via Stop Module Req?"=FALSE, "Wait for Module to stop?"=FALSE, "ModuleAdmin"=refnum} ("Stop Argument"), Variant=w217) -> (data=w213:T5, error out=w200:errorcluster)
        n78 = Unbundle By Name(w213) -> ("ModuleAdmin"=w207:refnum<class "ModuleAdmin.lvclass">)
        n79 = property class="ModuleAdmin.lvclass"(reference=w207, error in=w200) -> (error out=w201:errorcluster, "Accessors:ModuleName"=w205:string, "Accessors:Module ID"=w204:i32, "Accessors:CloneRegRef"=w203:refnum<data-value>)  [unwired: 1 out]
        n80 = Get Date/Time In Seconds() -> (seconds since 1Jan1904=w220:timestamp)
        n81 = Get Date/Time String(date format (0)=enum16{"short", "long", "abbreviated"}."short", seconds (now)=w220, want seconds? (F)=TRUE) -> (time string=w222:string)  [unwired: 1 out]
        n82 = Format Into String(format string="%s: %s:%d %s \\r", initial string=w216, error in=w201, w222, w205, w204, "Stopping") -> (resulting string=w215:string, error out=w199:errorcluster)
        n83 = control-ref of="Select Module"() -> (w212:refnum<vi>)
        n84 = call "UpdateSelectRing.vi"("error in (no error)"=w199, "CloneRegRef"=w203, "Ring Refnum"=w212) -> ("error out"=w209:errorcluster, "ActiveModules"=w211:string[], "Module Ring Value"=w210:i32)  [unwired: 6 in]
        n85 = local write "Active Modules (Array)"(w211) -> ()
      }
      event User Event {
        # "Time stamp and add the Status message to the log"
        # "The data types for the broadcast messages\nare in PublicAPI/Broadcasts"
        n86 = event-data() -> ("Data"=w232:variant)  [unwired: 1 in]
        n87 = Variant To Data(error in=w233, type="" ("clStatUpdate"), Variant=w232) -> (data=w225:string, error out=w223:errorcluster)
        n88 = Get Date/Time In Seconds() -> (seconds since 1Jan1904=w230:timestamp)
        n89 = Get Date/Time String(date format (0)=enum16{"short", "long", "abbreviated"}."short", seconds (now)=w230, want seconds? (F)=TRUE) -> (time string=w226:string)  [unwired: 1 out]
        n90 = Format Into String(format string="%s: %s \\r", initial string=w235, error in=w223, w226, w225) -> (resulting string=w229:string)  [unwired: 1 out]
      }
      event User Event {
        n91 = event-data() -> ("Data"=w242:variant)  [unwired: 1 in]
        n92 = Variant To Data(error in=w243, type=cluster{string, "Cluster":T1} {"", "Cluster"={"Configuration Mode"=enum."Constant Voltage (DC)", "Phases"=[]}}, Variant=w242) -> (data=w238:cluster{string, "Cluster":T1}, error out=w240:errorcluster)
        n93 = Unbundle(w238) -> ("Cluster"=w237:T1)  [unwired: 1 out]
        n94 = local write "Cluster"(w237) -> ()
      }
      event User Event {
        n95 = event-data() -> ("ModuleID"=w246:i32, "Data"=w256:variant)  [unwired: 1 in]
        n96 = Variant To Data(error in=w258, type=cluster{string, "Data":variant} {"", "Data"=variant}, Variant=w256) -> (data=w254:cluster{string, "Data":variant}, error out=w257:errorcluster)
        n97 = Unbundle(w254) -> (w248:string, "Data"=w253:variant)
        n98 = Equal?(x="CHROMAAC", y=w248) -> (x = y?=w251:bool)
        n99 = Equal?(x=w248, y="CHROMADC") -> (x = y?=w277:bool)
        n100 = Equal?(x="PPS", y=w248) -> (x = y?=w291:bool)
        n101 = Equal?(x="NHRDC", y=w248) -> (x = y?=w284:bool)
        n102 = Number To Decimal String(number=w246) -> (decimal integer string=w265:string)  [unwired: 1 in]
        n103 = Number To Decimal String(number=w246) -> (decimal integer string=w264:string)  [unwired: 1 in]
        n104 = Number To Decimal String(number=w246) -> (decimal integer string=w263:string)  [unwired: 1 in]
        n105 = Number To Decimal String(number=w246) -> (decimal integer string=w268:string)  [unwired: 1 in]
        n106 = control-ref of="Chroma AC"() -> (w290:refnum<vi>)
        n107 = control-ref of="Chroma DC"() -> (w276:refnum<vi>)
        n108 = control-ref of="PacificPower"() -> (w281:refnum<vi>)
        n109 = control-ref of="NHRDC"() -> (w280:refnum<vi>)
        n110 = call "DatatoGraphNHR.vi"("Caption"=w268, "ExtractData"=w284, "error in (no error)"=w257, "Array 2"=u32[] [0, 1, 0, 0], "Data"=w253, "NHRDC WaveformChart 2"=w280) -> ("error out"=w282:errorcluster, "Array"=→"NHRDC":waveform(sgl)[], "Incorrect DataType?"=→"NHRDC Incorrect Data Type?":bool)  [unwired: 3 in]
        n111 = call "DatatoGraphChroma.vi"("Caption.Text"=w265, "Boolean"=w251, "error in (no error)"=w257, "Array 2"=u32[] [0, 1, 0, 0], "Data"=w253, "WaveformChart in"=w290) -> ("error out"=w286:errorcluster, "OutputString"=w275:string, "Array"=→"Chroma AC":waveform(dbl)[], "Incorrect DataType?"=→"Chroma AC Incorrect Data Type?":bool)  [unwired: 2 in]
        n112 = call "DatatoGraphChroma.vi"("Caption.Text"=w264, "Boolean"=w277, "error in (no error)"=w257, "Array 2"=u32[] [0, 1, 0, 0], "Data"=w253, "WaveformChart in"=w276) -> ("error out"=w278:errorcluster, "OutputString"=w269:string, "Array"=→"Chroma DC":waveform(dbl)[], "Incorrect DataType?"=→"Chroma DC Incorrect Data Type?":bool)  [unwired: 2 in]
        n113 = call "DatatoGraphPP.vi"("Caption.Text"=w263, "ExtractData"=w291, "error in (no error)"=w257, "Array 2"=u32[] [0, 1, 0, 0, 1], "Data"=w253, "PacificPowerWavefromChart 2"=w281) -> ("error out"=w292:errorcluster, "Array"=→"PacificPower":waveform(dbl)[], "Incorrect DataType?"=→"PP Incorrect Data Type?":bool)  [unwired: 3 in]
        n114 = call "OutputChromaError.vi"("error in (no error)"=w286, "Chroma Output String"=w275, "Initial Message String"=w274) -> ("error out"=w273:errorcluster, "Output String"=w271:string)  [unwired: 7 in]
        n115 = call "OutputChromaError.vi"("error in (no error)"=w273, "Chroma Output String"=w269, "Initial Message String"=w271) -> ("error out"=w272:errorcluster, "Output String"=w270:string)  [unwired: 7 in]
        n116 = Merge Errors(w272, w278, w292, w282) -> (w293:errorcluster)
      }
      event User Event {
        # "#CodeNeeded\nThis is a very crude error handler\nA better error handler will be needed"
        # "The data types for the broadcast messages\nare in PublicAPI/Broadcasts"
        n117 = event-data() -> ("ModuleID"=w300:i32, "Data"=w304:variant)  [unwired: 1 in]
        n118 = Number To Decimal String(number=w300) -> (decimal integer string=w299:string)  [unwired: 1 in]
        n119 = Variant To Data(error in=w303, type=errorcluster {"status"=FALSE, "code"=0, "source"=""} ("Cluster"), Variant=w304) -> (data=w296:errorcluster, error out=w302:errorcluster)
        n120 = call <vilib>:"General Error Handler.vi"("[error source] (\" \")"=w299, "error in (no error)"=w296) -> ()  [unwired: 9 in, 5 out]
      }
      event User Event {
        n121 = event-data() -> ("Data"=w309:variant)  [unwired: 1 in]
        n122 = Variant To Data(error in=w307, type=path "" ("Path"), Variant=w309) -> (data=→"Path":path, error out=w306:errorcluster)
      }
      event User Event {
        # "Time stamp and add the DidInit message to the log"
        n123 = event-data() -> ("Data"=w327:variant)  [unwired: 1 in]
        n124 = call "IniFiles.vi"("error in"=w316, "iniKey"="Type", "name or relative path"="..\\..\\UserFiles\\Plugins\\AcPwr") -> ("error out"=w335:errorcluster, "Types"=w336:string[], "IniFilePaths"=w337:path[])  [unwired: 6 in]
        n125 = property on="Plugin Type" class="Ring (strict)"(error in=w335, "Strings []"=w336) -> (error out=w315:errorcluster)  [unwired: 1 in, 1 out]
        n126 = Bundle By Name(cluster=T2 {"PluginIniFilePaths"=[]} ("TestInfo"), "PluginIniFilePaths"=w337) -> (w334:T2)
        n127 = call "TestInfo.vi"("Set (f)"=TRUE, "TestInfo 2"=w334) -> ()  [unwired: 9 in, 1 out]
        n128 = Variant To Data(error in=w315, type=T4 {"Init?"=FALSE, "ModuleAdmin"=refnum} ("clDidInit"), Variant=w327) -> (data=w313:T4, error out=w314:errorcluster)
        n129 = Unbundle By Name(w313) -> ("ModuleAdmin"=w326:refnum<class "ModuleAdmin.lvclass">)
        n130 = property class="ModuleAdmin.lvclass"(reference=w326, error in=w314) -> (error out=w321:errorcluster, "Accessors:ModuleName"=w319:string, "Accessors:Module ID"=w318:i32)  [unwired: 1 out]
        n131 = Get Date/Time In Seconds() -> (seconds since 1Jan1904=w331:timestamp)
        n132 = Get Date/Time String(date format (0)=enum16{"short", "long", "abbreviated"}."short", seconds (now)=w331, want seconds? (F)=TRUE) -> (time string=w320:string)  [unwired: 1 out]
        n133 = Format Into String(format string="%s: %s:%d %s \\r", initial string=w325, error in=w321, w320, w319, w318, "INI File Loaded") -> (resulting string=w323:string, error out=w324:errorcluster)
      }
    }
    "Status Log" <- w31
    n134 = call <vilib>:"Simple Error Handler.vi"("error in (no error)"=w33) -> ("error out"=w25:errorcluster)  [unwired: 4 in, 4 out]
    n135 = property on="Status Log" class="Str"(error in=w25, "Text.Scroll Position"=-1) -> (error out=w24:errorcluster)  [unwired: 1 in, 1 out]
  }
  n136 = Unregister For Events(event registration refnum=w2, error in=w3) -> ()  [unwired: 1 out]
